vi "POS_Folder name from filename.vi"(11 "File Path In":path) -> (3 "Folder Path Out":path)   [LabVIEW 2012]
doc: "SciScan 1.2 160622"
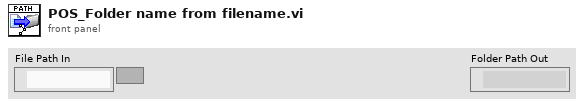
[diagram p1: front panel]
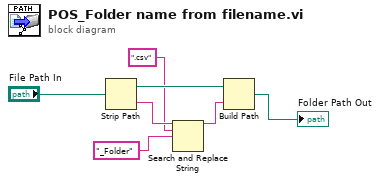
[diagram p0: block diagram]
diagram:
  n1 = Strip Path(path="File Path In") -> (stripped path=w6:path, name=w5:string)
  n2 = Search and Replace String(input string=w5, search string=".csv", replace string="_Folder" ("replace string (\"\")")) -> (result string=w2:string)  [unwired: 5 in, 3 out]
  n3 = Build Path(base path=w6, name or relative path=w2) -> (appended path=→"Folder Path Out":path)
